vi "Read Network Master.vi"(8 "error in (no error)":errorcluster, 11 "Modbus master in":refnum<class "Modbus Master.lvclass">) -> (0 "error out":errorcluster, 2 "network master":refnum<class "Network Master.lvclass">, 3 "Modbus master out":refnum<class "Modbus Master.lvclass">)   [LabVIEW 2018, in "Modbus Master.lvclass"]
doc: "This VI is an accessor for the <B>network master</B> stored in the Modbus master instance. This accessor can be used as a property node. This network master is used by the Modbus instance to communicate on the physical bus."
uses:
  Modbus Master.lvclass
  Network Master.lvclass
  Modbus Master.lvclass/Modbus Master.ctl
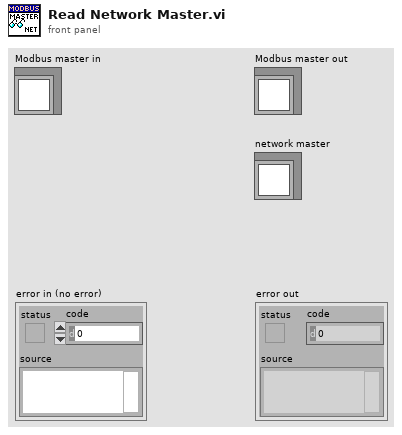
[diagram p1: front panel]
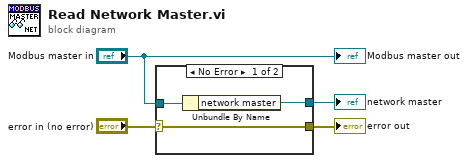
[diagram p0: block diagram]
diagram:
  n1 = case shown="No Error" "error in (no error)" {
    selector: "error in (no error)" -> [w5 w8]
    tunnel: "Modbus master in" -> [w7 _]
    tunnel: [w6 _] -> w3
    tunnel: [w5 w8] -> w1
    frame No Error {
      n2 = Unbundle By Name(w7) -> ("network master"=w6:refnum<class "Network Master.lvclass">)
    }
    frame Error {
    }
  }
  "error out" <- w1
  "network master" <- w3
  "Modbus master out" <- "Modbus master in"
